vi "takeHalfBack.vi"(1 "gain":dbl, 2 "targetRPM":dbl, 3 "actualRPM":dbl) -> (0 "motorOutput":dbl)   [LabVIEW 2012]
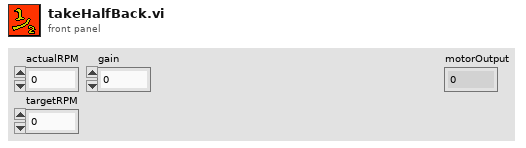
[diagram p1: front panel]
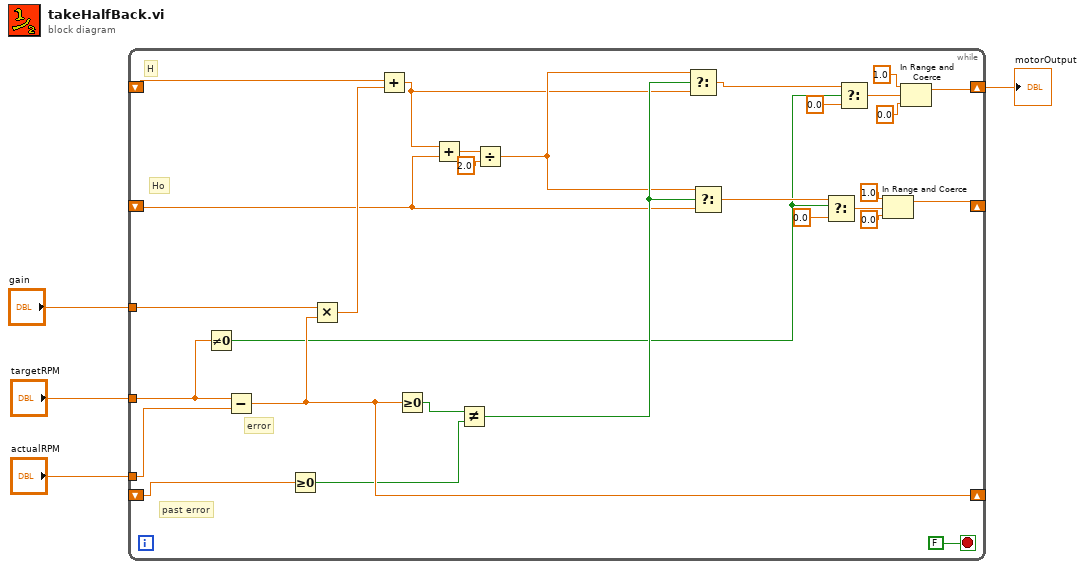
[diagram p0: block diagram]
diagram:
  n1 = while {
    tunnel: "targetRPM" -> [w32]
    tunnel: "actualRPM" -> [w33]
    tunnel: "gain" -> [w31]
    shift-right: [w25] -> _
    shift-left: _ -> [w24]
    shift-right: [w20] -> w1
    shift-left: _ -> [w19]
    shift-right: [w7] -> _
    shift-left: _ -> [w6]
    stop <- FALSE stop-if-true
    # "past error"
    # "Ho"
    # "H"
    # "error"
    n2 = Not Equal To 0?(x=w32) -> (x != 0?=w12:bool)
    n3 = Subtract(x=w32, y=w33) -> (x-y=w25:dbl)
    n4 = Greater Or Equal To 0?(x=w24) -> (x >= 0?=w22:bool)
    n5 = Multiply(x=w31, y=w25) -> (x*y=w30:dbl)
    n6 = Add(x=w19, y=w30) -> (x+y=w11:dbl)
    n7 = Greater Or Equal To 0?(x=w25) -> (x >= 0?=w23:bool)
    n8 = Add(x=w11, y=w6) -> (x+y=w18:dbl)
    n9 = Not Equal?(x=w23, y=w22) -> (x != y?=w16:bool)
    n10 = Divide(x=w18, y=2.0) -> (x/y=w15:dbl)
    n11 = Select(t=w15, s=w16, f=w11) -> (s? t:f=w21:dbl)
    n12 = Select(t=w15, s=w16, f=w6) -> (s? t:f=w14:dbl)
    n13 = Select(t=w14, s=w12, f=0.0) -> (s? t:f=w10:dbl)
    n14 = Select(t=w21, s=w12, f=0.0) -> (s? t:f=w27:dbl)
    n15 = In Range and Coerce(upper limit=1.0, x=w10, lower limit=0.0) -> (coerced(x)=w7:dbl)  [unwired: 1 out]
    n16 = In Range and Coerce(upper limit=1.0, x=w27, lower limit=0.0) -> (coerced(x)=w20:dbl)  [unwired: 1 out]
  }
  "motorOutput" <- w1
